vi "10Ax4 בחירת בדיקות עבור ממסר.vi"(0 "Enable":bool=TRUE, 5 "error in (no error)":errorcluster) -> (11 "בחר הכל":bool, 12 "בדיקת מפל מתח בין דקי הממסר תחת עומס":bool, 14 "בדיקת זמן מיתוג הממסר":bool, 15 "בדיקת צריכת זרם של סליל הפיקוד":bool, 16 "בדיקת מתח שחרור של סליל פיקוד ללא עומס":bool, 17 "בדיקת מתח תפיסה של סליל פיקוד ללא עומס":bool, 18 "OK":bool, 19 "error out":errorcluster)   [LabVIEW 2015]
doc: "Displays a standard dialog box that prompts users to enter information, such as a user name and password.\n--------------------\n\nThis Express VI is configured as follows:\n\nMessage to Display to the User:15A בחירת בדיקות עבור הממסר\nThe inputs are: \nCheckbox: בדיקת מתח תפיסה של סליל פיקוד ללא עומס\nCheckbox: בדיקת מתח שחרור של סליל פיקוד ללא עומס\nCheckbox: בדיקת צריכת זרם של סליל הפיקוד\nCheckbox: בדיקת זמן מיתוג הממסר\nCheckbox: בדיקת זמן ניתוק הממסר\nCheckbox: בדיקת מפל מתח בין דקי הממסר תחת עומס\nCheckbox: בחר הכל"
panel:
  in  "בחר הכל":bool
  in  "בדיקת מפל מתח בין דקי הממסר תחת עומס":bool
  in  "בדיקת זמן מיתוג הממסר":bool
  in  "בדיקת צריכת זרם של סליל הפיקוד":bool
  in  "בדיקת מתח שחרור של סליל פיקוד ללא עומס":bool
  in  "בדיקת מתח תפיסה של סליל פיקוד ללא עומס":bool
  in  "Cancel":bool
  in  "OK2":bool
  in  "OK1":bool
  # "10Ax4 בחירת בדיקות עבור ממסר"
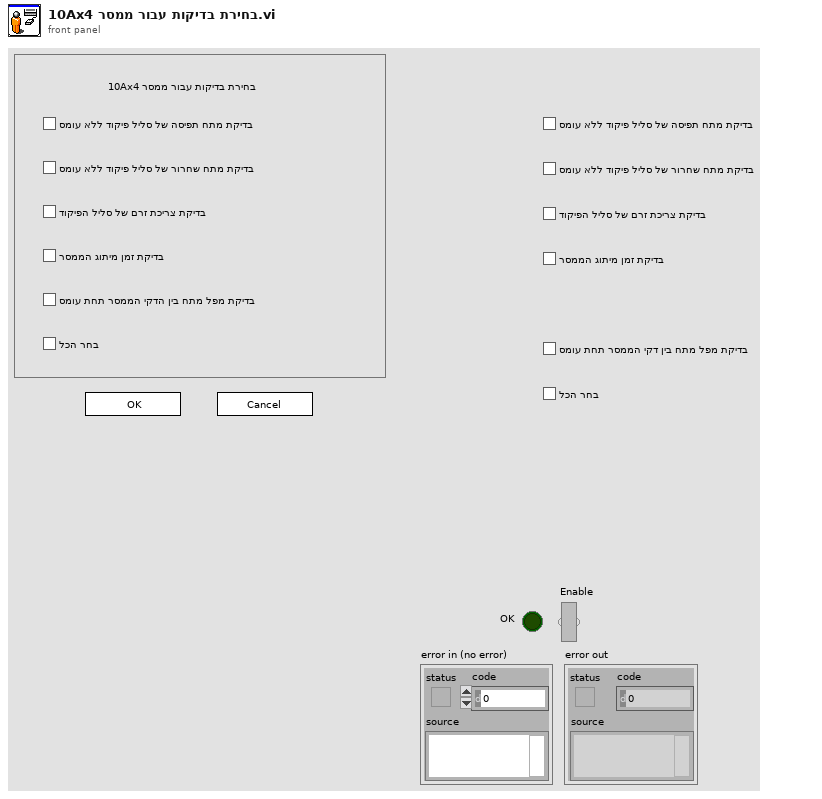
[diagram p1: front panel]
types:
  T1 = cluster{"Input Name":string, "Input Data Type":i32}[]
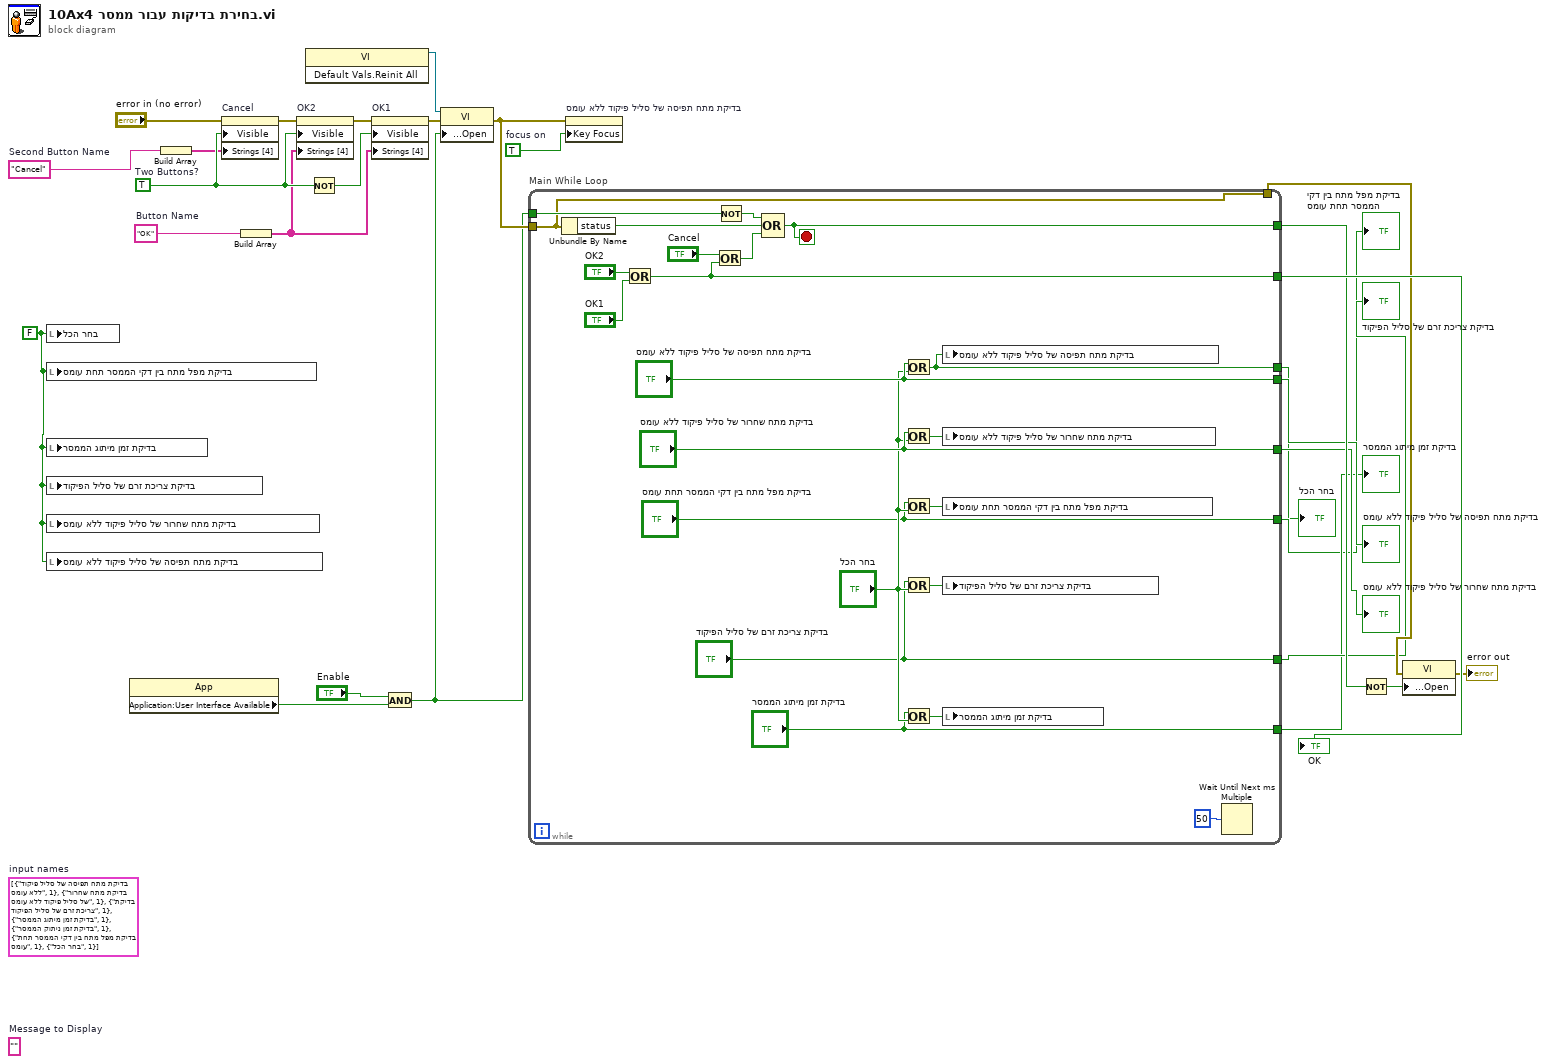
[diagram p0: block diagram]
diagram:
  w1 = FALSE ("בחר הכל")
  w7 = TRUE  # focus on
  (unwired) T1 [{"Input Name"="בדיקת מתח תפיסה של סליל פיקוד ללא עומס", "Input Data Type"=1}, {"Input Name"="בדיקת מתח שחרור של סליל פיקוד ללא עומס", "Input Data Type"=1}, {"Input Name"="בדיקת צריכת זרם של סליל הפיקוד", "Input Data Type"=1}, {"Input Name"="בדיקת זמן מיתוג הממסר", "Input Data Type"=1}, {"Input Name"="בדיקת זמן ניתוק הממסר", "Input Data Type"=1}, {"Input Name"="בדיקת מפל מתח בין דקי הממסר תחת עומס", "Input Data Type"=1}, {"Input Name"="בחר הכל", "Input Data Type"=1}]  # input names
  w20 = "Cancel"  # Second Button Name
  w18 = "OK"  # Button Name
  (unwired) ""  # Message to Display
  w28 = TRUE  # Two Buttons?
  n1 = local write "בחר הכל"(w1) -> ()
  n2 = local write "בדיקת מפל מתח בין דקי הממסר תחת עומס"(w1) -> ()
  n3 = local write "בדיקת זמן מיתוג הממסר"(w1) -> ()
  n4 = local write "בדיקת צריכת זרם של סליל הפיקוד"(w1) -> ()
  n5 = local write "בדיקת מתח שחרור של סליל פיקוד ללא עומס"(w1) -> ()
  n6 = local write "בדיקת מתח תפיסה של סליל פיקוד ללא עומס"(w1) -> ()
  n7 = property class="App"() -> ("Application:User Interface Available"=w10:bool)  [unwired: 2 in, 2 out]
  n8 = Build Array(w20) -> (w21:string[])
  n9 = property on="Cancel" class="Bool"(error in="error in (no error)", "Visible"=w28, "Strings [4]"=w21) -> (error out=w25:errorcluster)  [unwired: 1 in, 1 out]
  n10 = Build Array(w18) -> (w19:string[])
  n11 = property on="OK2" class="Bool"(error in=w25, "Visible"=w28, "Strings [4]"=w19) -> (error out=w24:errorcluster)  [unwired: 1 in, 1 out]
  n12 = invoke class="VI" method="Default Vals.Reinit All"() -> (reference out=w9:refnum<vi>)  [unwired: 3 in, 2 out]
  n13 = Not(x=w28) -> (.not. x?=w26:bool)
  n14 = property on="OK1" class="Bool"(error in=w24, "Visible"=w26, "Strings [4]"=w19) -> (error out=w17:errorcluster)  [unwired: 1 in, 1 out]
  n15 = And(x="Enable", y=w10) -> (x .and. y?=w11:bool)
  n16 = property class="VI"(reference=w9, error in=w17, "Front Panel Window:Open"=w11) -> (error out=w16:errorcluster)  [unwired: 1 out]
  n17 = while "Main While Loop" {
    tunnel: [w47] -> w27
    tunnel: w11 -> [w45]
    tunnel: [w43] -> w22
    tunnel: w16 -> [w42]
    tunnel: [w42] -> w14
    tunnel: ["בדיקת מתח תפיסה של סליל פיקוד ללא עומס"] -> w8
    tunnel: ["בדיקת מתח שחרור של סליל פיקוד ללא עומס"] -> w6
    tunnel: ["בדיקת צריכת זרם של סליל הפיקוד"] -> w5
    tunnel: ["בדיקת זמן מיתוג הממסר"] -> w4
    tunnel: ["בדיקת מפל מתח בין דקי הממסר תחת עומס"] -> w3
    tunnel: [w39] -> w2
    stop <- w43 stop-if-true
    n18 = Unbundle By Name(w42) -> ("status"=w40:bool)
    n19 = Or(x="OK2", y="OK1") -> (x .or. y?=w47:bool)
    n20 = Or(x="Cancel", y=w47) -> (x .or. y?=w41:bool)
    n21 = Not(x=w45) -> (.not. x?=w44:bool)
    n22 = Compound Arithmetic op=OR(w44, w40, w41) -> (w43:bool)
    n23 = Or(x="בדיקת מתח תפיסה של סליל פיקוד ללא עומס", y="בחר הכל") -> (x .or. y?=w39:bool)
    n24 = Or(x="בדיקת מתח שחרור של סליל פיקוד ללא עומס", y="בחר הכל") -> (x .or. y?=w36:bool)
    n25 = Or(x="בדיקת מפל מתח בין דקי הממסר תחת עומס", y="בחר הכל") -> (x .or. y?=w30:bool)
    n26 = Or(x="בדיקת צריכת זרם של סליל הפיקוד", y="בחר הכל") -> (x .or. y?=w29:bool)
    n27 = Or(x="בדיקת זמן מיתוג הממסר", y="בחר הכל") -> (x .or. y?=w31:bool)
    n28 = local write "בדיקת מתח תפיסה של סליל פיקוד ללא עומס"(w39) -> ()
    n29 = local write "בדיקת מתח שחרור של סליל פיקוד ללא עומס"(w36) -> ()
    n30 = local write "בדיקת מפל מתח בין דקי הממסר תחת עומס"(w30) -> ()
    n31 = local write "בדיקת צריכת זרם של סליל הפיקוד"(w29) -> ()
    n32 = local write "בדיקת זמן מיתוג הממסר"(w31) -> ()
    n33 = Wait Until Next ms Multiple(millisecond multiple=u32 50) -> ()  [unwired: 1 out]
  }
  "OK" <- w27
  "בדיקת מתח תפיסה של סליל פיקוד ללא עומס" <- w8
  "בדיקת מתח שחרור של סליל פיקוד ללא עומס" <- w6
  "בדיקת צריכת זרם של סליל הפיקוד" <- w5
  "בדיקת זמן מיתוג הממסר" <- w4
  "בדיקת מפל מתח בין דקי הממסר תחת עומס" <- w3
  "בחר הכל" <- w2
  n34 = property on="בדיקת מתח תפיסה של סליל פיקוד ללא עומס" class="Bool (strict)"(error in=w16, "Key Focus"=w7) -> ()  [unwired: 1 in, 2 out]
  n35 = Not(x=w22) -> (.not. x?=w23:bool)
  n36 = property class="VI"(error in=w14, "Front Panel Window:Open"=w23) -> (error out=→"error out":errorcluster)  [unwired: 1 in, 1 out]
